vi "Init Data.vi"(8 "error in (no error)":errorcluster, 10 "Data Object":refnum<class "Factory Plugin Framework.lvclass">, 11 "File Parsing Interface in":refnum<class "File Parsing Interface.lvclass">) -> (0 "error out":errorcluster, 3 "File Parsing Interface out":refnum<class "File Parsing Interface.lvclass">)   [LabVIEW 2018, in "File Parsing Interface.lvlib" / "File Parsing Interface.lvclass"]
uses:
  File Parsing Interface.lvclass
  Plugins/FPF.lvlibp/Factory Plugin Framework.lvclass
  File Parsing Interface.lvclass/File Parsing Interface.ctl
  Accessors/File to Parse/Read File to Parse.vi
  Accessors/File to Parse/Write File to Parse.vi
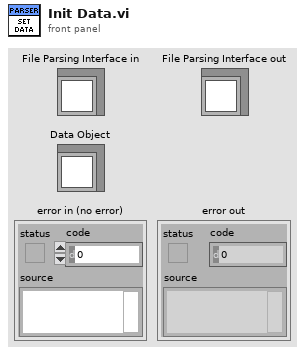
[diagram p1: front panel]
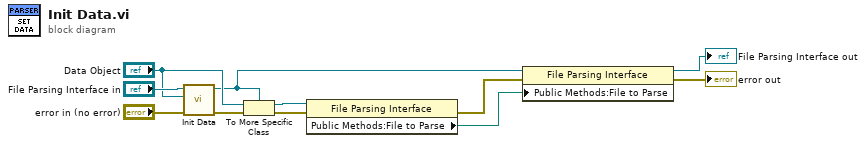
[diagram p0: block diagram]
diagram:
  n1 = call-parent "Init Data.vi"("error in (no error)"="error in (no error)", "Data Object"="Data Object", "Factory Plugin Framework in"="File Parsing Interface in") -> ("error out"=w11:errorcluster, "Factory Plugin Framework out"=w2:refnum<class "File Parsing Interface.lvclass">)  [unwired: 7 in]
  n2 = To More Specific Class(target class=w2, reference="Data Object", error in=w11) -> (specific class reference=w5:refnum<class "File Parsing Interface.lvclass">, error out=w8:errorcluster)
  n3 = property class="File Parsing Interface"(reference=w5, error in=w8) -> (error out=w6:errorcluster, "Public Methods:File to Parse"=w1:path)  [unwired: 1 out]
  n4 = property class="File Parsing Interface"(reference=w2, error in=w6, "Public Methods:File to Parse"=w1) -> (reference out=→"File Parsing Interface out":refnum<class "File Parsing Interface.lvclass">, error out=→"error out":errorcluster)
